vi "EOL CAN_Get_Motor_Hall_Position (2).vi"(11 "NetworkObjHandle":u32) -> (1 "Hall Position":u16, 2 "TxRx Data":string[][](array[string]), 3 "Response Good?":bool)   [LabVIEW 2012]
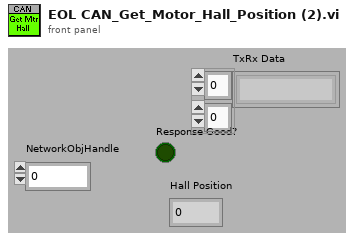
[diagram p1: front panel]
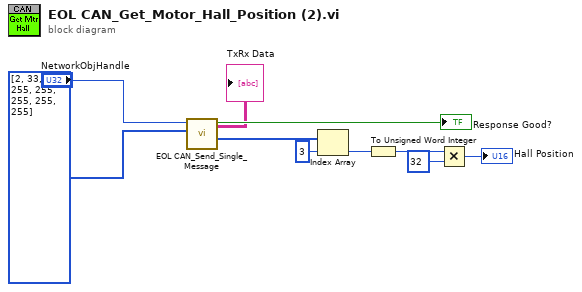
[diagram p0: block diagram]
diagram:
  n1 = call "EOL CAN_Send_Single_Message.vi"("Read Session in"=u8[] [2, 33, 99, 255, 255, 255, 255, 255] ("Transmit Data"), "Write Session in"="NetworkObjHandle") -> ("Rx Message"=w7:u8[], "Response Good?"=→"Response Good?":bool, "TxRx Data"=→"TxRx Data":string[][])  [unwired: 5 in, 2 out]
  n2 = Index Array(array=w7, index=3) -> (element=w5:u8)
  n3 = To Unsigned Word Integer(number=w5) -> (unsigned 16bit integer=w2:u16)
  n4 = Multiply(x=w2, y=u16 32) -> (x*y=→"Hall Position":u16)
